vi "Select Waveforms Dialog.vi"(5 "Selected Channel Refs":T1[](array[typedef]) format="%.0x", 6 "Expand GUIDs":string[](array[string]), 7 "Channel Label":string="System Channels", 8 "error in (no error)":errorcluster, 9 "Custom Filter":refnum<k24>, 10 "Filter":u8(ring) items=["K_CHAN_R", "K_CHAN_W", "K_CHAN_RW", "K_CHAN_VOLT", "K_CHAN_FAULT", "K_ALL", "K_CUSTOM", "K_CHAN_R_VIS", "K_CHAN_W_VIS", "K_CHAN_RW_VIS", "K_CHAN_VOLT_VIS", "K_CHAN_FAULT_VIS", "K_WAVE", "K_WAVE_VIS", "K_WAVE_DBL", "K_WAVE_CDB", "K_WAVE_DBL_VIS", "K_WAVE_CDB_VIS"], 11 "Start Item Ref":T1=18446744073709551615 format="%.0x") -> (0 "error out":errorcluster, 1 "Canceled":bool, 3 "Channels":string[](array[string]))   [LabVIEW 2015, in "Waveform Data Logger System Explorer.lvlib"]
uses:
  Waveform Data Logger System Explorer.lvlib
  <vilib>/NI Veristand/Custom Device API/Custom Device Item Ref.ctl
  NationalInstruments.VeriStand.SystemStorageUI
  NationalInstruments.VeriStand.SystemStorage
  <userlib>/_OpenG.lib/array/array.llb/Remove Duplicates from 1D Array (String)__ogtk.vi
  <vilib>/NI VeriStand/Custom Device API/Custom Device API.lvlib
panel:
  in  "OK":bool
  in  "Cancel":bool
  in  "System Channels":refnum<k24>(container)
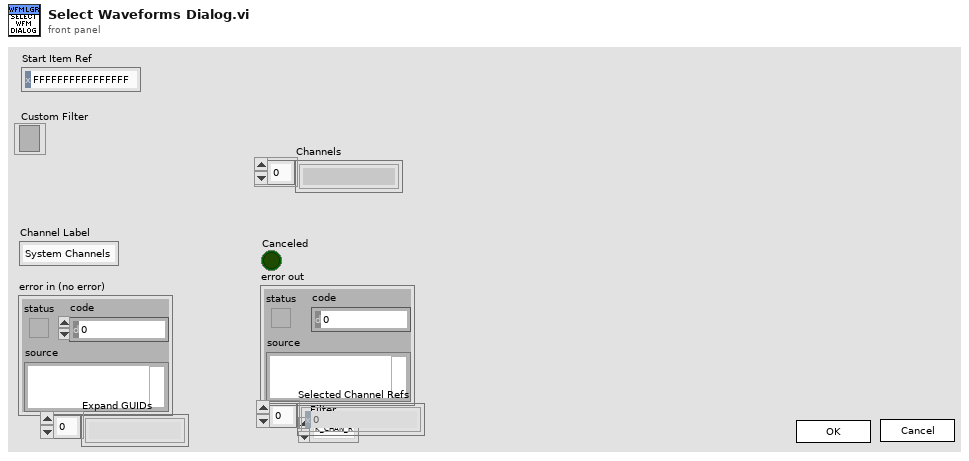
[diagram p1: front panel]
types:
  T1 = typedef "Custom Device API.lvlib/Custom Device Item Ref.ctl" = u64
  T2 = cluster{"Shut Down":bool, "Error":errorcluster, "Root":refnum<k24>, "Cancel":bool, "MapTree":cluster{"Ref":refnum<k24>, "Filter":refnum<k24>}, "Channels":string[]}
  T3 = typedef "Custom Device API.lvlib/Custom Device Pointer.ctl" = refnum<k24>
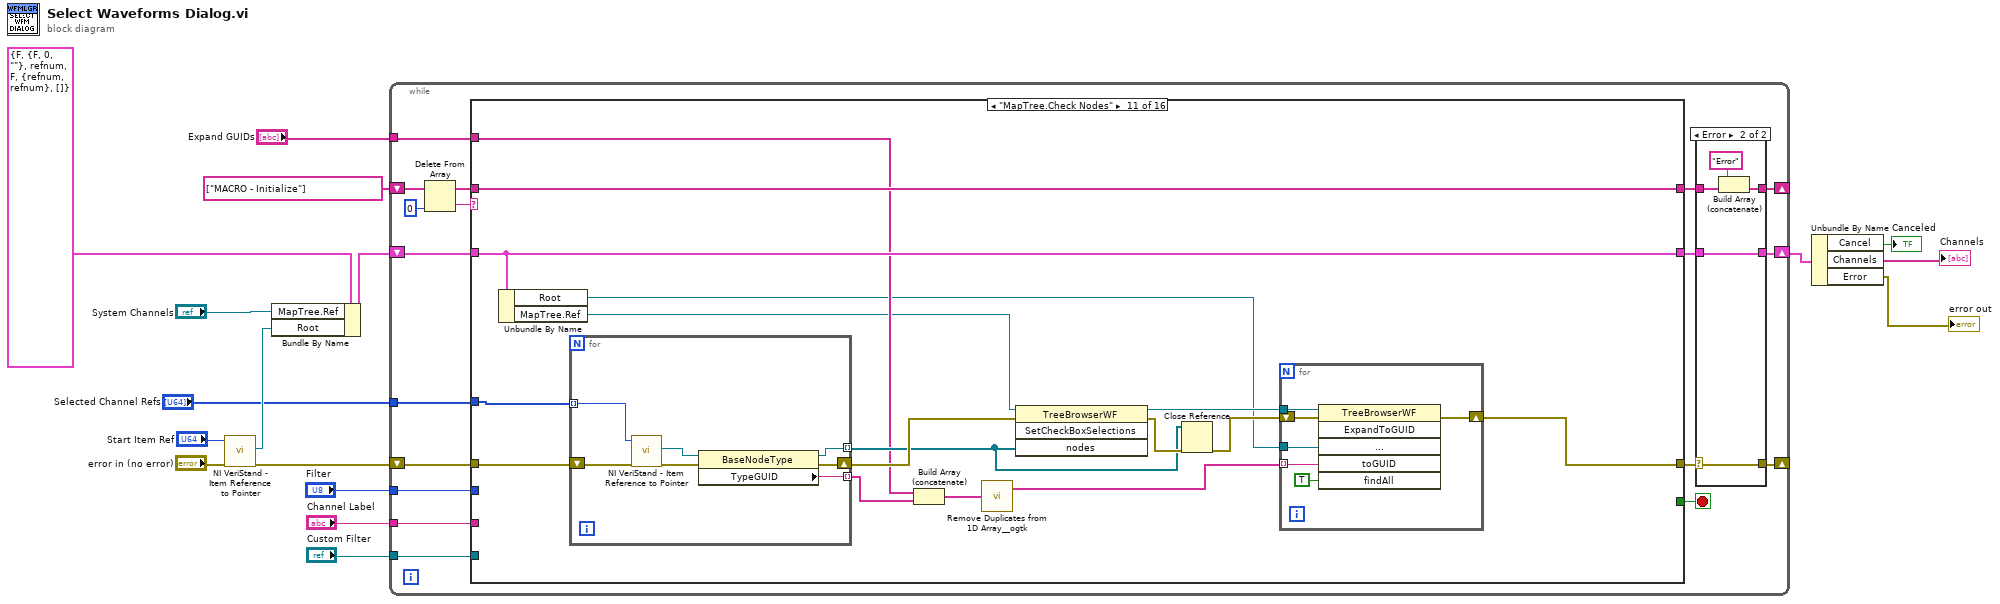
[diagram p0: block diagram]
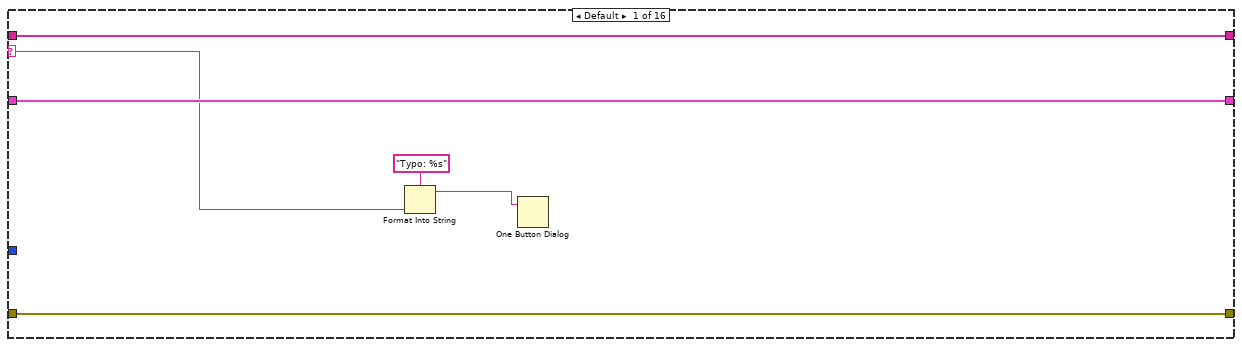
[diagram p3: hidden frame]
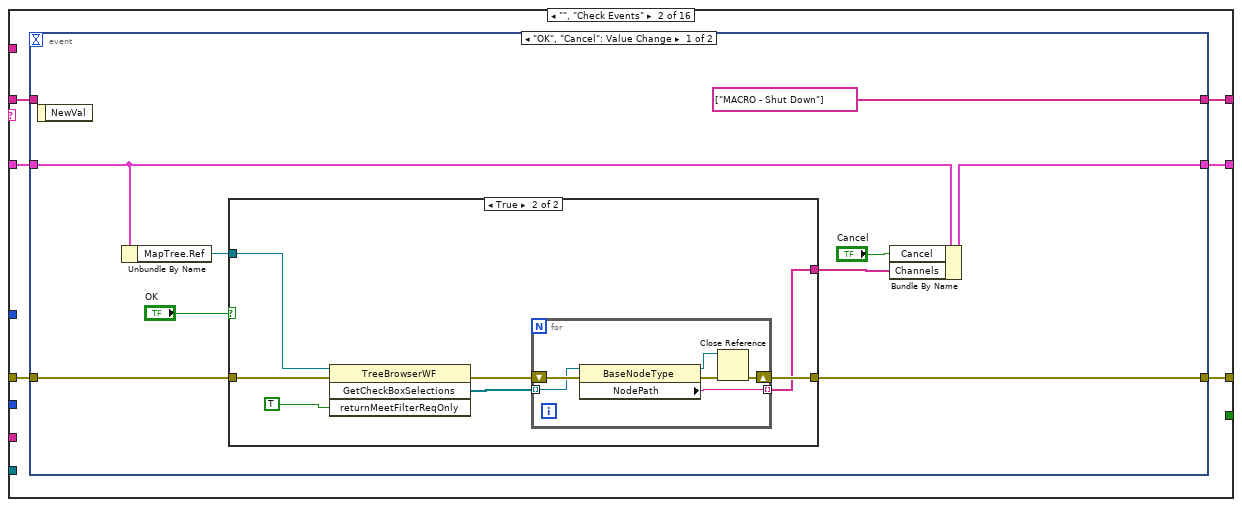
[diagram p4: hidden frame]
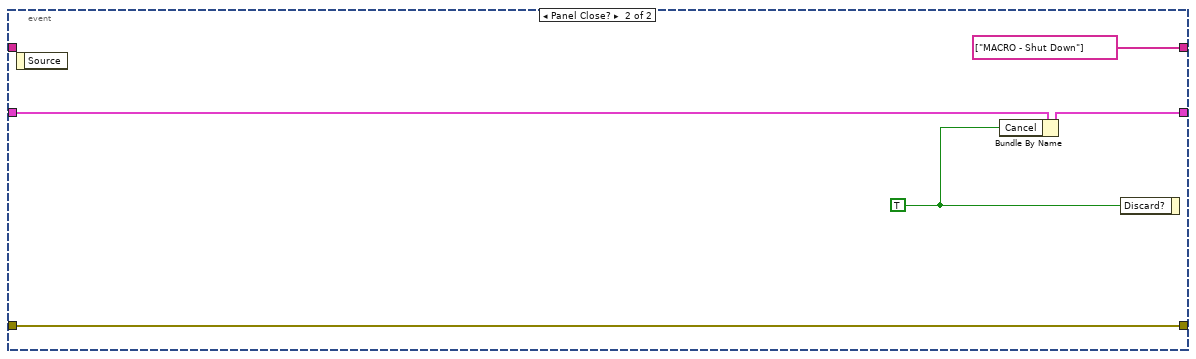
[diagram p6: hidden frame]
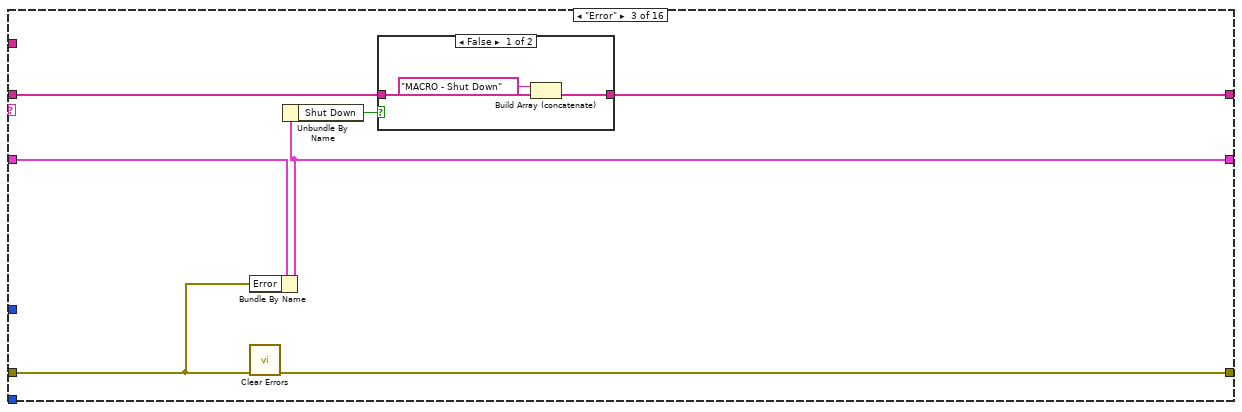
[diagram p7: hidden frame]
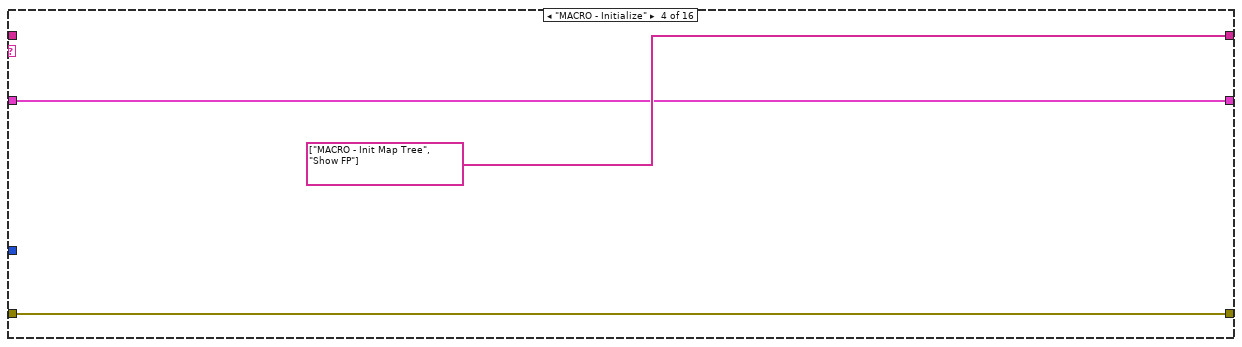
[diagram p9: hidden frame]
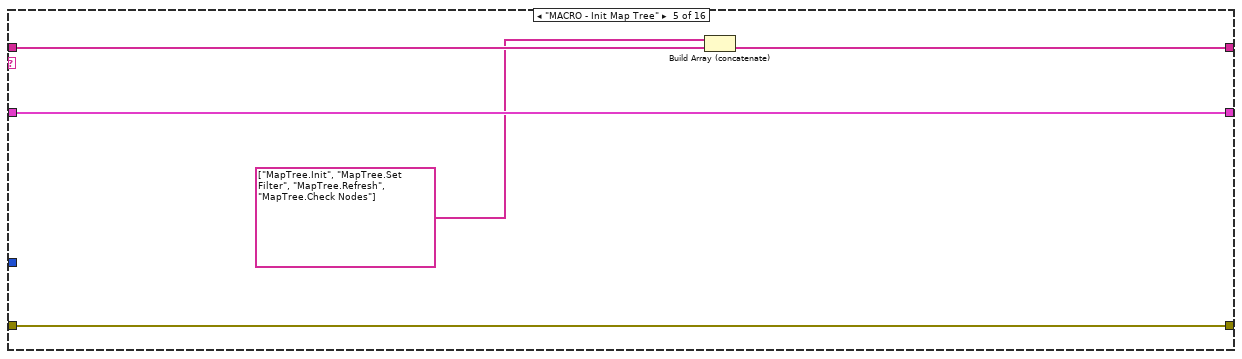
[diagram p10: hidden frame]
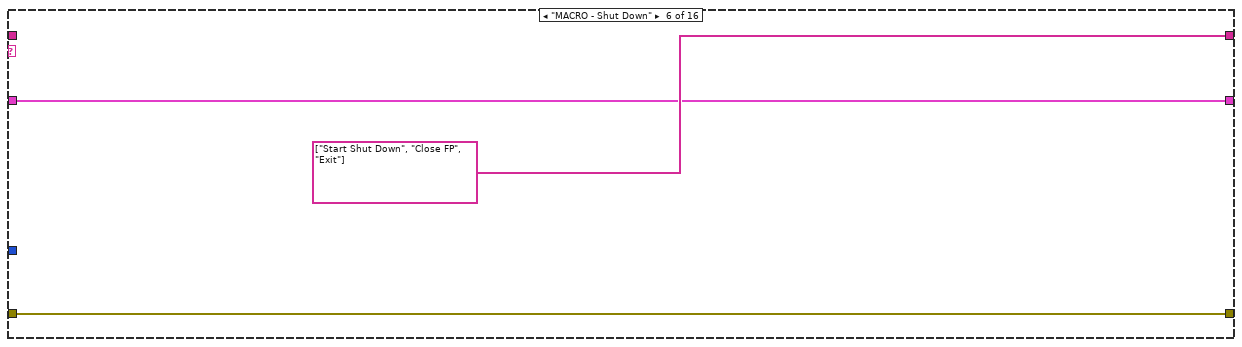
[diagram p11: hidden frame]
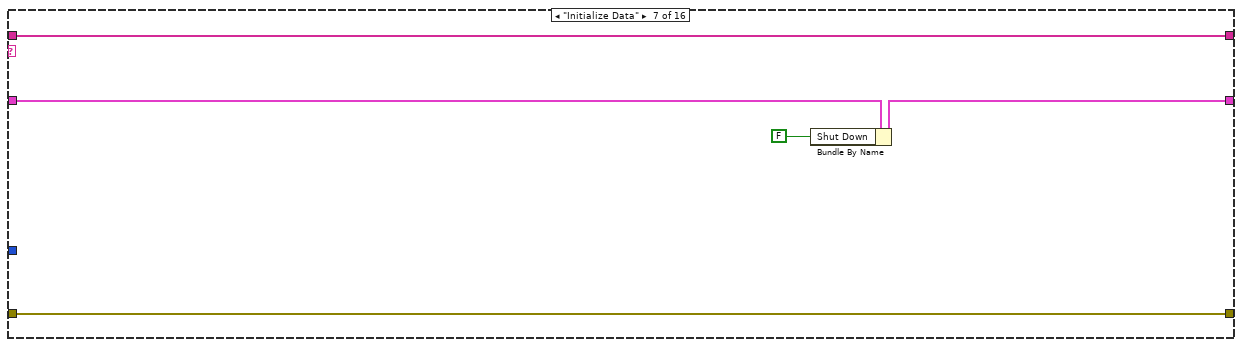
[diagram p12: hidden frame]
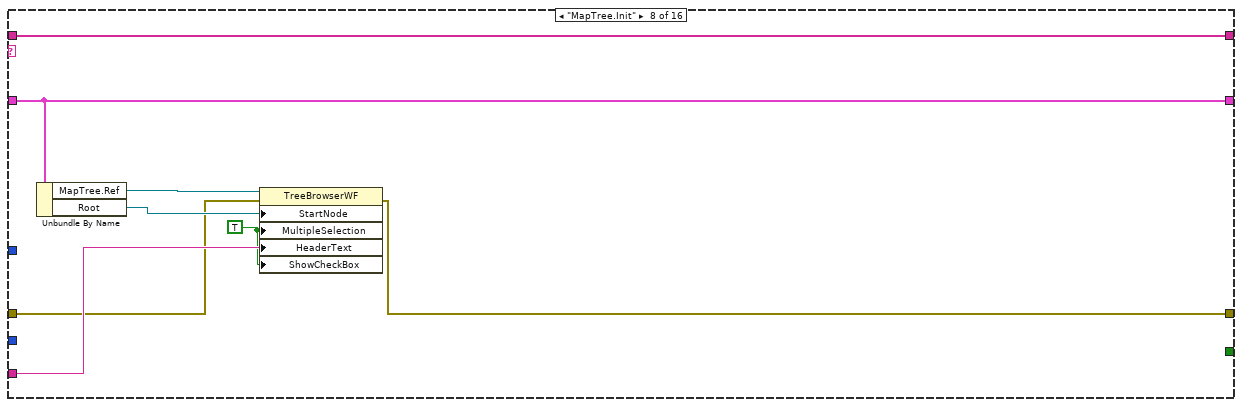
[diagram p13: hidden frame]
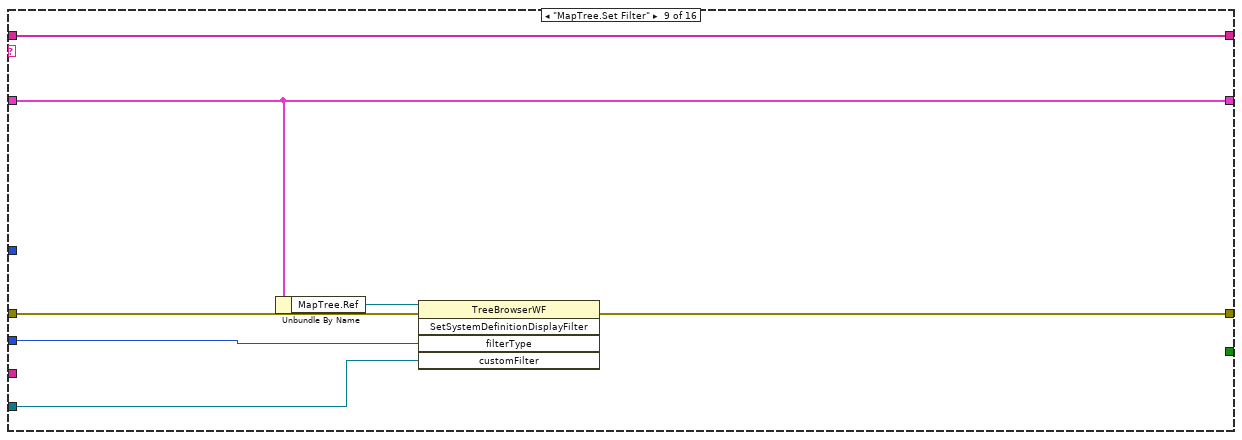
[diagram p14: hidden frame]
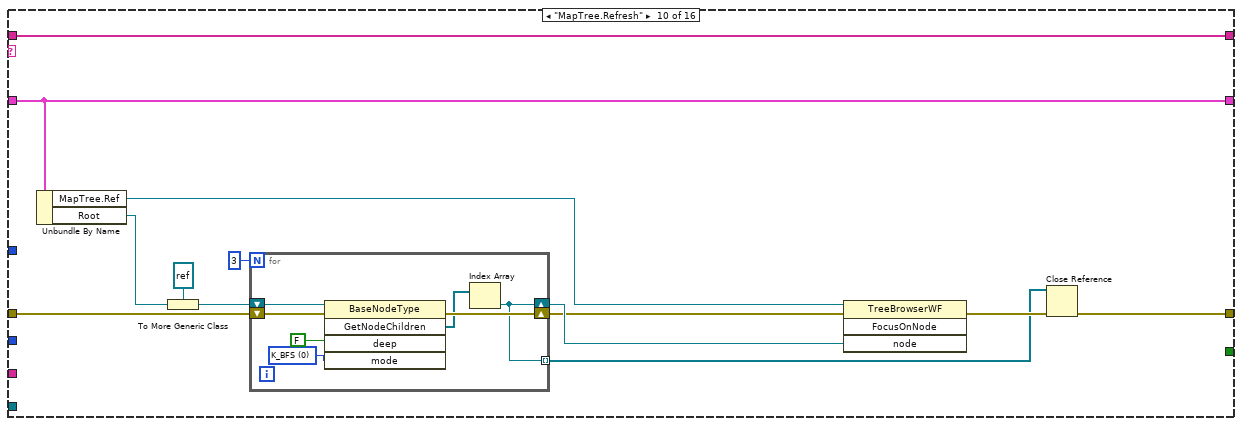
[diagram p15: hidden frame]
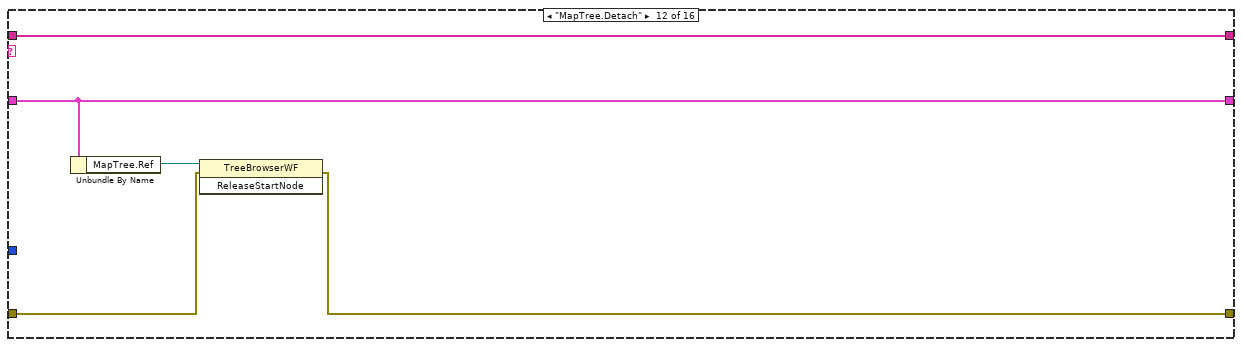
[diagram p16: hidden frame]
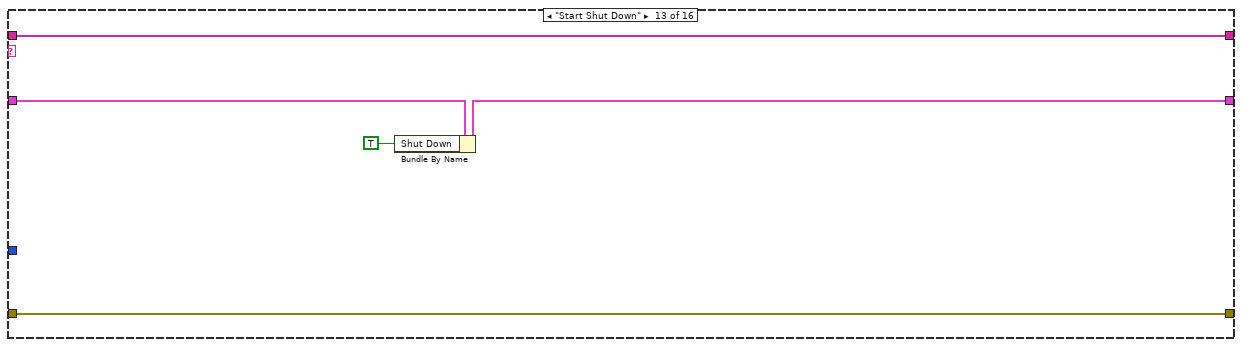
[diagram p17: hidden frame]
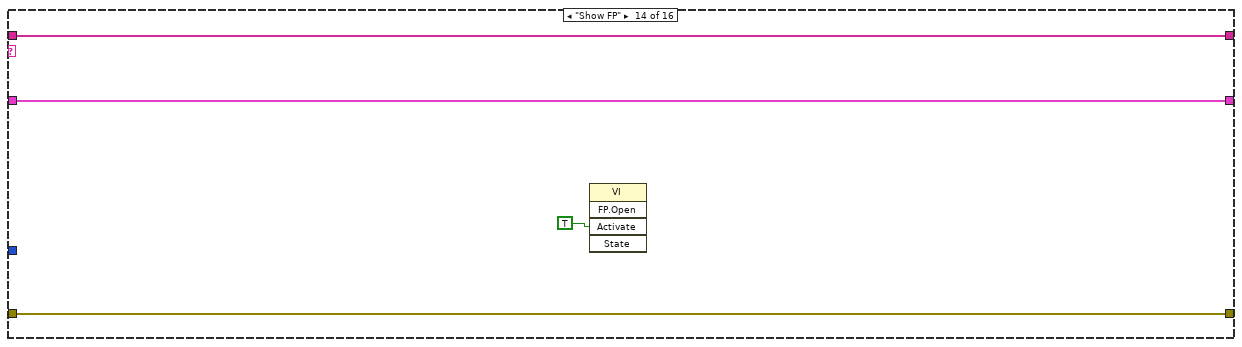
[diagram p18: hidden frame]
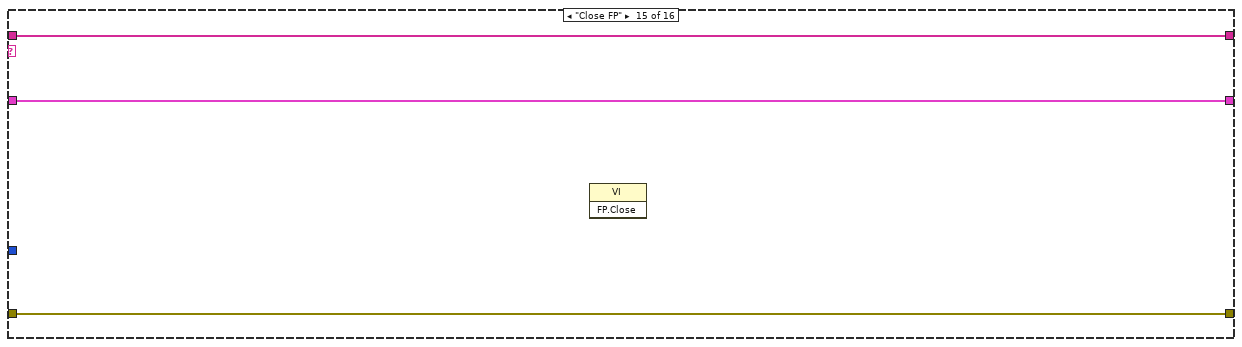
[diagram p19: hidden frame]
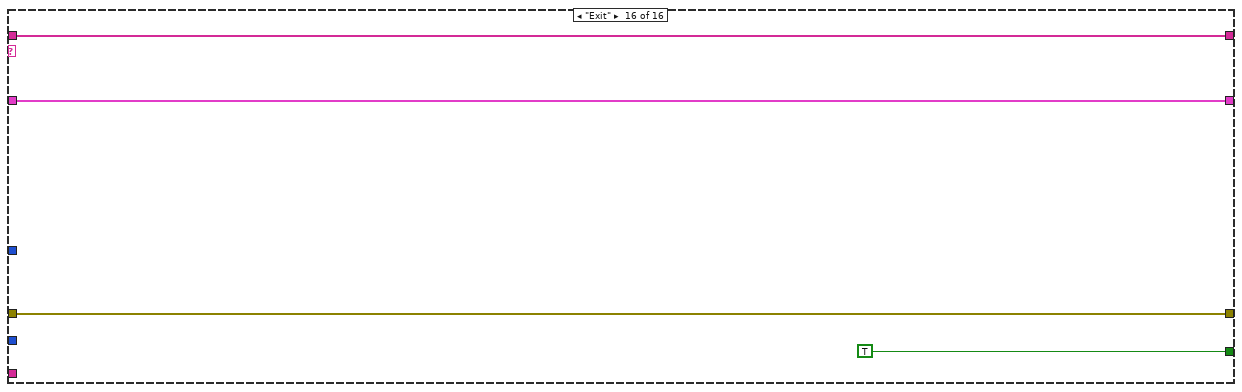
[diagram p20: hidden frame]
diagram:
  n1 = call <vilib>:"NI VeriStand - Item Reference to Pointer.vi"("error in (no error)"="error in (no error)", "Item Ref in"="Start Item Ref") -> ("error out"=w5:errorcluster, "Node Pointer"=w3:T3)  [unwired: 6 in, 2 out]
  n2 = Bundle By Name(cluster=T2 {"Shut Down"=FALSE, "Error"={"status"=FALSE, "code"=0, "source"=""}, "Root"=refnum, "Cancel"=FALSE, "MapTree"={"Ref"=refnum, "Filter"=refnum}, "Channels"=[]} ("State Data"), "MapTree.Ref"="System Channels", "Root"=w3) -> (w14:T2)
  n3 = while {
    shift-right: [w25] -> _
    shift-left: string[] ["MACRO - Initialize"] -> [w35]
    shift-right: [w27] -> _
    shift-left: w5 -> [w31]
    shift-right: [w24] -> w11
    shift-left: w14 -> [w29]
    tunnel: "Channel Label" -> [w22]
    tunnel: "Filter" -> [w21]
    tunnel: "Custom Filter" -> [w20]
    tunnel: "Selected Channel Refs" -> [w19]
    tunnel: "Expand GUIDs" -> [w18]
    stop <- w30 stop-if-true
    n4 = Delete From Array(array=w35, index=0) -> (deleted portion=w32:string, array with subset deleted=w33:string[])  [unwired: 1 in]
    n5 = case shown="\"MapTree.Check Nodes\"" w32 {
      selector: w32 -> [w45 _ _ _ _ _ _ _ _ _ _ _ _ _ _ _]
      tunnel: w33 -> [w49 w55 w87 _ w102 _ w110 w118 w125 w138 w161 w179 w180 w188 w191 w195]
      tunnel: [w49 w50 w86 string[] ["MACRO - Init Map Tree", "Show FP"] ("array") w99 string[] ["Start Shut Down", "Close FP", "Exit"] ("array") w110 w118 w125 w138 w161 w179 w180 w188 w191 w195] -> w26
      tunnel: [w48 w53 w84 w97 w101 w105 w109 w111 w123 w128 w152 w175 w184 w187 w190 w194] -> w28
      tunnel: w31 -> [w48 w52 w85 w97 w101 w105 w109 w112 w121 w136 w158 w176 w184 w187 w190 w194]
      tunnel: [_ _ _ _ _ _ _ _ _ _ _ _ _ _ _ TRUE] -> w30
      tunnel: w29 -> [w47 w54 w90 w95 w100 w103 w106 w117 w122 w137 w160 w178 w183 w186 w189 w192]
      tunnel: [w47 w51 w89 w95 w100 w103 w108 w117 w122 w137 w160 w178 w182 w186 w189 w192] -> w23
      tunnel: w22 -> [_ _ _ _ _ _ _ w114 _ _ _ _ _ _ _ _]
      tunnel: w21 -> [_ _ _ _ _ _ _ _ w120 _ _ _ _ _ _ _]
      tunnel: w20 -> [_ _ _ _ _ _ _ _ w119 _ _ _ _ _ _ _]
      tunnel: w19 -> [_ _ _ _ _ _ _ _ _ _ w159 _ _ _ _ _]
      tunnel: w18 -> [_ _ _ _ _ _ _ _ _ _ w151 _ _ _ _ _]
      frame Default {
        n6 = Format Into String(format string="Typo: %s", w45) -> (resulting string=w44:string)  [unwired: 2 in, 1 out]
        n7 = One Button Dialog(message=w44) -> ()  [unwired: 1 in, 1 out]
      }
      frame "", "Check Events" {
        n8 = event shown="[0] \"OK\", \"Cancel\": Value Change" {
          selector: _ -> [_ _]
          dyn-events: _ -> [_ _]
          timeout: _ -> [_ _]
          tunnel: [w57 w83] -> w53
          tunnel: w52 -> [w59 w83]
          tunnel: [w63 w80] -> w51
          tunnel: w54 -> [w61 w82]
          tunnel: w55 -> [_ _]
          tunnel: [string[] ["MACRO - Shut Down"] string[] ["MACRO - Shut Down"]] -> w50
          event "OK", "Cancel": Value Change {
            n9 = event-data() -> ()  [unwired: 1 in, 1 out]
            n10 = Unbundle By Name(w61) -> ("MapTree.Ref"=w60:refnum<k24>)
            n11 = case shown="True" "OK" {
              tunnel: w60 -> [_ w72]
              tunnel: w59 -> [w65 w71]
              tunnel: [_ w66] -> w58
              tunnel: [w65 w67] -> w57
              frame False {
              }
              frame True {
                n12 = invoke class="TreeBrowserWF" method="GetCheckBoxSelections"(reference=w72, error in=w71, "returnMeetFilterReqOnly"=TRUE) -> (error out=w69:errorcluster, "GetCheckBoxSelections"=w68:refnum<k24>[])  [unwired: 1 in, 2 out]
                n13 = for {
                  shift-right: [w73] -> w67
                  shift-left: w69 -> [w78]
                  tunnel: w68 -> [w77] mode=indexing
                  tunnel: [w76] -> w66 mode=indexing
                  n14 = property class="BaseNodeType"(reference=w77, error in=w78) -> (reference out=w74:refnum<k24>, error out=w75:errorcluster, "NodePath"=w76:string)
                  n15 = Close Reference(reference=w74, error in (no error)=w75) -> (error out=w73:errorcluster)
                }
              }
            }
            n16 = Bundle By Name(cluster=w61, "Cancel"="Cancel", "Channels"=w58) -> (w63:T2)
          }
          event Panel Close? {
            w79 = TRUE ("Discard?")
            n17 = event-data() -> ()  [unwired: 1 in, 1 out]
            n18 = Bundle By Name(cluster=w82, "Cancel"=w79) -> (w80:T2)
            n19 = event-data("Discard?"=w79) -> ()  [unwired: 1 in, 1 out]
          }
        }
      }
      frame "Error" {
        n20 = Bundle By Name(cluster=w90, "Error"=w85) -> (w89:T2)
        n21 = call <vilib>:"Clear Errors.vi"("error in (no error)"=w85) -> ("error out"=w84:errorcluster)  [unwired: 5 in, 1 out]
        n22 = Unbundle By Name(w89) -> ("Shut Down"=w88:bool)
        n23 = case shown="False" w88 {
          tunnel: w87 -> [w92 w94]
          tunnel: [w91 w94] -> w86
          frame False {
            n24 = Build Array (concatenate)("MACRO - Shut Down", w92) -> (w91:string[])
          }
          frame True {
            # "Do not interrupt a shut down sequence. This can cause an infinite loop."
          }
        }
      }
      frame "MACRO - Initialize" {
      }
      frame "MACRO - Init Map Tree" {
        n25 = Build Array (concatenate)(string[] ["MapTree.Init", "MapTree.Set Filter", "MapTree.Refresh", "MapTree.Check Nodes"] ("array"), w102) -> (w99:string[])
      }
      frame "MACRO - Shut Down" {
      }
      frame "Initialize Data" {
        n26 = Bundle By Name(cluster=w106, "Shut Down"=FALSE) -> (w108:T2)
      }
      frame "MapTree.Init" {
        w113 = TRUE ("MultipleSelection")
        n27 = Unbundle By Name(w117) -> ("MapTree.Ref"=w116:refnum<k24>, "Root"=w115:refnum<k24>)
        n28 = property class="TreeBrowserWF"(reference=w116, error in=w112, "StartNode"=w115, "MultipleSelection"=w113, "HeaderText"=w114, "ShowCheckBox"=w113) -> (error out=w111:errorcluster)  [unwired: 1 out]
      }
      frame "MapTree.Set Filter" {
        n29 = Unbundle By Name(w122) -> ("MapTree.Ref"=w124:refnum<k24>)
        n30 = invoke class="TreeBrowserWF" method="SetSystemDefinitionDisplayFilter"(reference=w124, error in=w121, "filterType"=w120, "customFilter"=w119) -> (error out=w123:errorcluster)  [unwired: 1 in, 4 out]
      }
      frame "MapTree.Refresh" {
        n31 = Unbundle By Name(w137) -> ("MapTree.Ref"=w126:refnum<k24>, "Root"=w135:refnum<k24>)
        n32 = To More Generic Class(target class=refnum<k24> refnum, reference=w135) -> (generic class reference=w133:refnum<k24>)
        n33 = for {
          N: 3 -> [_]
          shift-right: [w139] -> w132
          shift-left: w133 -> [w142]
          shift-right: [w145] -> w127
          shift-left: w136 -> [w141]
          tunnel: [w139] -> w129 mode=indexing
          w143 = 0 items=["K_BFS", "K_DFS", "K_CHILDONLY", "K_UP"] ("mode")
          n34 = invoke class="BaseNodeType" method="GetNodeChildren"(reference=w142, error in=w141, "deep"=FALSE, "mode"=w143) -> (error out=w145:errorcluster, "GetNodeChildren"=w140:refnum<k24>[])  [unwired: 1 in, 3 out]
          n35 = Index Array(array=w140) -> (element=w139:refnum<k24>)  [unwired: 1 in]
        }
        n36 = invoke class="TreeBrowserWF" method="FocusOnNode"(reference=w126, error in=w127, "node"=w132) -> (error out=w130:errorcluster)  [unwired: 1 in, 3 out]
        n37 = Close Reference(reference=w129, error in (no error)=w130) -> (error out=w128:errorcluster)
      }
      frame "MapTree.Check Nodes" {
        n38 = Unbundle By Name(w160) -> ("Root"=w147:refnum<k24>, "MapTree.Ref"=w146:refnum<k24>)
        n39 = for {
          tunnel: w159 -> [w173] mode=indexing
          shift-right: [w170] -> w157
          shift-left: w158 -> [w174]
          tunnel: [w169] -> w155 mode=indexing
          tunnel: [w168] -> w149 mode=indexing
          n40 = call <vilib>:"NI VeriStand - Item Reference to Pointer.vi"("error in (no error)"=w174, "Item Ref in"=w173) -> ("error out"=w171:errorcluster, "Node Pointer"=w172:T3)  [unwired: 6 in, 2 out]
          n41 = property class="BaseNodeType"(reference=w172, error in=w171) -> (reference out=w169:T3, error out=w170:errorcluster, "TypeGUID"=w168:string)
        }
        n42 = Build Array (concatenate)(w151, w149) -> (w150:string[])
        n43 = call-poly <userlib>:"Remove Duplicates from 1D Array__ogtk.vi"("Input Array"=w150) -> ("Output Array"=w148:string[])  [unwired: 1 out]
        n44 = invoke class="TreeBrowserWF" method="SetCheckBoxSelections"(reference=w146, error in=w157, "nodes"=w155) -> (reference out=w154:refnum<k24>, error out=w156:errorcluster)  [unwired: 1 in, 2 out]
        n45 = Close Reference(reference=w155, error in (no error)=w156) -> (error out=w153:errorcluster)
        n46 = for {
          tunnel: w154 -> [w167]
          shift-right: [w165] -> w152
          shift-left: w153 -> [w166]
          tunnel: w147 -> [w164]
          tunnel: w148 -> [w163] mode=indexing
          n47 = invoke class="TreeBrowserWF" method="ExpandToGUID"(reference=w167, error in=w166, "startNode"=w164, "toGUID"=w163, "findAll"=TRUE) -> (error out=w165:errorcluster)  [unwired: 1 in, 5 out]
        }
      }
      frame "MapTree.Detach" {
        n48 = Unbundle By Name(w178) -> ("MapTree.Ref"=w177:refnum<k24>)
        n49 = invoke class="TreeBrowserWF" method="ReleaseStartNode"(reference=w177, error in=w176) -> (error out=w175:errorcluster)  [unwired: 1 in, 2 out]
      }
      frame "Start Shut Down" {
        n50 = Bundle By Name(cluster=w183, "Shut Down"=TRUE) -> (w182:T2)
      }
      frame "Show FP" {
        n51 = invoke class="VI" method="FP.Open"("Activate"=TRUE ("Activate?")) -> ()  [unwired: 4 in, 5 out]
      }
      frame "Close FP" {
        n52 = invoke class="VI" method="FP.Close"() -> ()  [unwired: 3 in, 3 out]
      }
      frame "Exit" {
      }
    }
    n53 = case shown="Error" w28 {
      selector: w28 -> [w38 w43]
      tunnel: [w38 w43] -> w27
      tunnel: w26 -> [w37 w41]
      tunnel: [w37 w40] -> w25
      tunnel: [w36 w42] -> w24
      tunnel: w23 -> [w36 w42]
      frame No Error {
      }
      frame Error {
        n54 = Build Array (concatenate)("Error", w41) -> (w40:string[])
      }
    }
  }
  n55 = Unbundle By Name(w11) -> ("Cancel"=→"Canceled":bool, "Channels"=→"Channels":string[], "Error"=→"error out":errorcluster)
